vi "generate channels from VI Terminals.vi"(8 "error in":errorcluster, 11 "VI Refnum":refnum<vi>) -> (0 "error out":errorcluster, 3 "channels":refnum<class "TBM channel.lvclass">[](array[class]))   [LabVIEW 2014, in "io configuration.lvclass"]
uses:
  io configuration.lvclass
  <vilib>/NI/Tag Bus Module Framework/channel/TBM channel.lvclass
  <vilib>/NI/Tag Bus Module Framework/channel/channel classification.ctl
  <vilib>/NI/Tag Bus/tag/Data Type.ctl
  <vilib>/NI/Tag Bus/tag/tag descriptor.lvclass
  <vilib>/Utility/VariantDataType/VariantType.lvlib
  <vilib>/fxp/LVFixedPointRepBitsTypeDef.ctl
  <vilib>/fxp/LVFixedPointRepRangeTypeDef.ctl
panel:
  out "Label.Text":string
  out "FXP Range":T1
  out "FXP Representation":T2
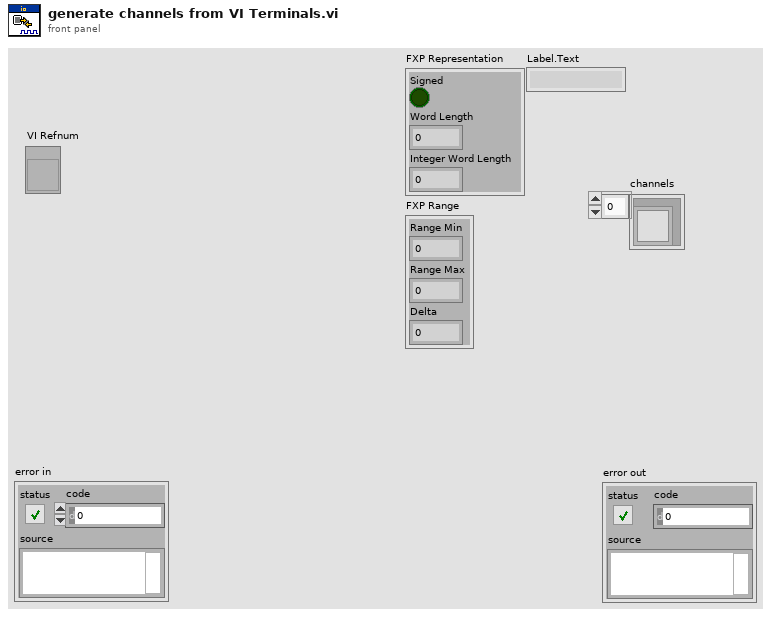
[diagram p1: front panel]
types:
  T1 = typedef "LVFixedPointRepRangeTypeDef.ctl" = cluster{"Range Min":dbl, "Range Max":dbl, "Delta":dbl}
  T2 = typedef "LVFixedPointRepBitsTypeDef.ctl" = cluster{"Signed":bool, "Word Length":u32, "Integer Word Length":i32}
  T3 = typedef "TBM channel.lvclass/channel classification.ctl" = enum16{"input data", "output data", "processing parameter", "processing result"}
  T4 = typedef "tag bus.lvlib/tag descriptor.lvclass/Data Type.ctl" = enum16{"Double", "Single", "I64", "I32", "I16", "I8", "U64", "U32", "U16", "U8", "Boolean", "String", "Array of Double", "Array of Single", "Array of I64", "Array of I32", "Array of I16", "Array of I8", "Array of U64", "Array of U32", "Array of U16", "Array of U8", "Array of Boolean", "Array of String"}
  T5 = typedef "VariantType.lvlib/Type.ctl" = enum8{"Invalid Type", "Void", "I8", "I16", "I32", "I64", "U8", "U16", "U32", "U64", "Single Float", "Double Float", "Extended Float", "Single Complex", "Double Complex", "Extended Complex", "Enum U8", "Enum U16", "Enum U32", "Enum U64", "Single Float With Unit", "Double Float With Unit", "Extended Float With Unit", "Single Complex with Unit", "Double Complex with Unit", "Extended Complex with Unit", "Boolean", "String", "Path", "Picture", "Tag", "Array", "Cluster", "Variant", "LV Variant", "Waveform", "Timestamp", "Digital Waveform", "Digital Data", "ExpressData", "Refnum", "External Data", "VI", "Poly VI", "LabVIEW Class Instance", "Fixed Point"}
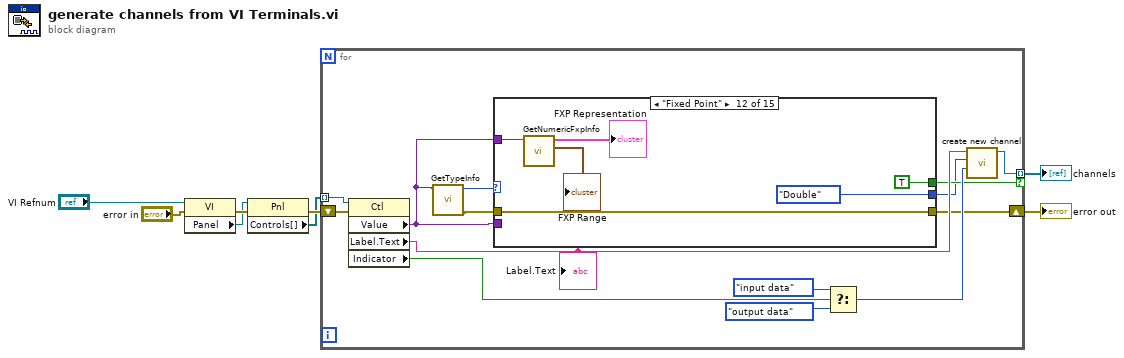
[diagram p0: block diagram]
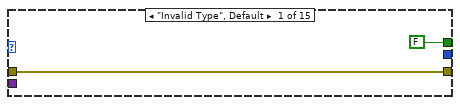
[diagram p2: hidden frame]
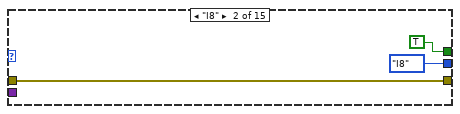
[diagram p3: hidden frame]
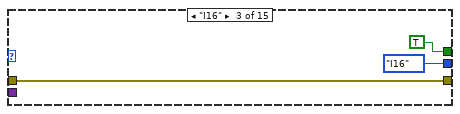
[diagram p4: hidden frame]
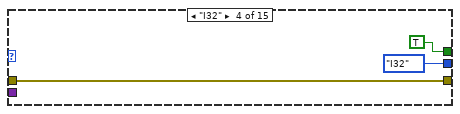
[diagram p5: hidden frame]
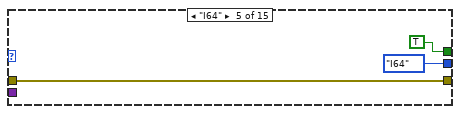
[diagram p6: hidden frame]
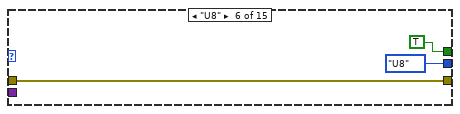
[diagram p7: hidden frame]
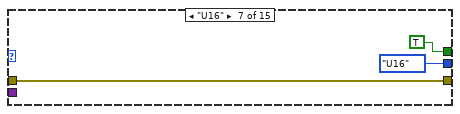
[diagram p8: hidden frame]
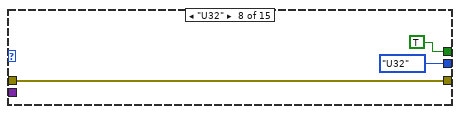
[diagram p9: hidden frame]
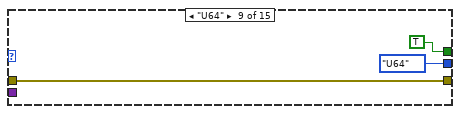
[diagram p10: hidden frame]
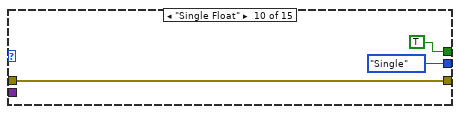
[diagram p11: hidden frame]
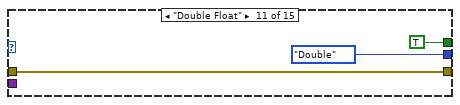
[diagram p12: hidden frame]
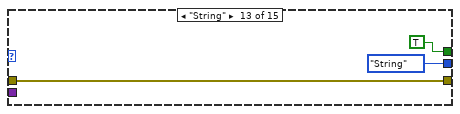
[diagram p13: hidden frame]
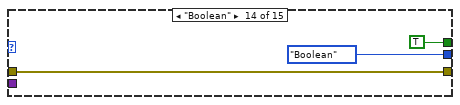
[diagram p14: hidden frame]
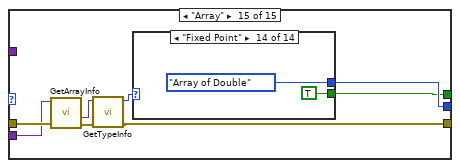
[diagram p15: hidden frame]
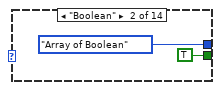
[diagram p17: hidden frame]
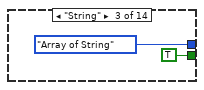
[diagram p18: hidden frame]
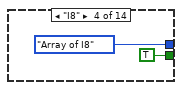
[diagram p19: hidden frame]
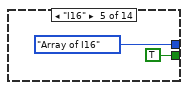
[diagram p20: hidden frame]
diagram:
  n1 = property class="VI"(reference="VI Refnum", error in="error in") -> (error out=w8:errorcluster, "Panel"=w7:refnum<vi>)  [unwired: 1 out]
  n2 = property class="Pnl"(reference=w7, error in=w8) -> (error out=w6:errorcluster, "Controls[]"=w5:refnum<vi>[])  [unwired: 1 out]
  n3 = for {
    shift-right: [w13] -> w2
    shift-left: w6 -> [w21]
    tunnel: w5 -> [w22] mode=indexing
    tunnel: [w20] -> w1 mode=indexing if=w15
    n4 = property class="Ctl"(reference=w22, error in=w21) -> ("Value"=w9:variant, "Label.Text"=w19:string, "Indicator"=w12:bool)  [unwired: 2 out]
    "Label.Text" <- w19
    n5 = call <vilib>:"GetTypeInfo.vi"("Variant"=w9) -> ("error out"=w10:errorcluster, "Type Enum"=w11:T5)  [unwired: 6 in, 3 out]
    n6 = case shown="\"Fixed Point\"" w11 {
      tunnel: w10 -> [w23 w25 w28 w31 w34 w37 w40 w43 w46 w49 w52 w58 w61 w64 w68]
      tunnel: w9 -> [_ _ _ _ _ _ _ _ _ _ _ _ _ _ w67]
      tunnel: [FALSE TRUE TRUE TRUE TRUE TRUE TRUE TRUE TRUE TRUE TRUE TRUE TRUE TRUE w73] -> w15
      tunnel: [_ Data_Type."I8" ("data type") Data_Type."I16" ("data type") Data_Type."I32" ("data type") Data_Type."I64" ("data type") Data_Type."U8" ("data type") Data_Type."U16" ("data type") Data_Type."U32" ("data type") Data_Type."U64" ("data type") Data_Type."Single" ("data type") Data_Type."Double" ("data type") Data_Type."Double" ("data type") Data_Type."String" ("data type") Data_Type."Boolean" ("data type") w74] -> w14
      tunnel: [w23 w25 w28 w31 w34 w37 w40 w43 w46 w49 w52 w58 w61 w64 w72] -> w13
      tunnel: w9 -> [_ _ _ _ _ _ _ _ _ _ _ w57 _ _ _]
      frame "Invalid Type", Default {
      }
      frame "I8" {
      }
      frame "I16" {
      }
      frame "I32" {
      }
      frame "I64" {
      }
      frame "U8" {
      }
      frame "U16" {
      }
      frame "U32" {
      }
      frame "U64" {
      }
      frame "Single Float" {
      }
      frame "Double Float" {
      }
      frame "Fixed Point" {
        n7 = call <vilib>:"GetNumericFxpInfo.vi"("Variant"=w57) -> ("FXP Range"=→"FXP Range":T1, "FXP Representation"=→"FXP Representation":T2)  [unwired: 7 in, 2 out]
      }
      frame "String" {
      }
      frame "Boolean" {
      }
      frame "Array" {
        n8 = call <vilib>:"GetArrayInfo.vi"("error in (no error)"=w68, "Variant"=w67) -> ("error out"=w70:errorcluster, "ArrayElement"=w69:variant)  [unwired: 6 in, 2 out]
        n9 = call <vilib>:"GetTypeInfo.vi"("error in (no error)"=w70, "Variant"=w69) -> ("error out"=w72:errorcluster, "Type Enum"=w71:T5)  [unwired: 5 in, 3 out]
        n10 = case shown="\"Fixed Point\"" w71 {
          tunnel: [_ Data_Type."Array of Boolean" ("data type") Data_Type."Array of String" ("data type") Data_Type."Array of I8" ("data type") Data_Type."Array of I16" ("data type") Data_Type."Array of I32" ("data type") Data_Type."Array of I64" ("data type") Data_Type."Array of U8" ("data type") Data_Type."Array of U16" ("data type") Data_Type."Array of U32" ("data type") Data_Type."Array of U64" ("data type") Data_Type."Array of Single" ("data type") Data_Type."Array of Double" ("data type") Data_Type."Array of Double" ("data type")] -> w74
          tunnel: [_ TRUE TRUE TRUE TRUE TRUE TRUE TRUE TRUE TRUE TRUE TRUE TRUE TRUE] -> w73
          frame "Invalid Type", Default {
          }
          frame "Boolean" {
          }
          frame "String" {
          }
          frame "I8" {
          }
          frame "I16" {
          }
          frame "I32" {
          }
          frame "I64" {
          }
          frame "U8" {
          }
          frame "U16" {
          }
          frame "U32" {
          }
          frame "U64" {
          }
          frame "Single Float" {
          }
          frame "Double Float" {
          }
          frame "Fixed Point" {
          }
        }
      }
    }
    n11 = Select(t=channel_classification."input data" ("channel classification"), s=w12, f=channel_classification."output data" ("channel classification")) -> (s? t:f=w16:T3)
    n12 = call <vilib>:"create new channel.vi"("channel classification"=w16, "data type"=w14, "channel name"=w19) -> ("channel"=w20:refnum<class "TBM channel.lvclass">)  [unwired: 8 in]
  }
  "error out" <- w2
  "channels" <- w1
